vi "step4 Solve.vi"(8 "error in (no error)":errorcluster, 11 "cube in":T1) -> (0 "error out":errorcluster, 1 "upper cross solved?":bool, 3 "cube out":T1)   [LabVIEW 2011]
doc: "Rotate cube as necessary so that the top middle piece matches the desired start colour.\n\nNo transformations are done in this VI, the operations are loaded on the the operation queue bus."
uses:
  Typedef/cube.ctl
  Typedef/face.ctl
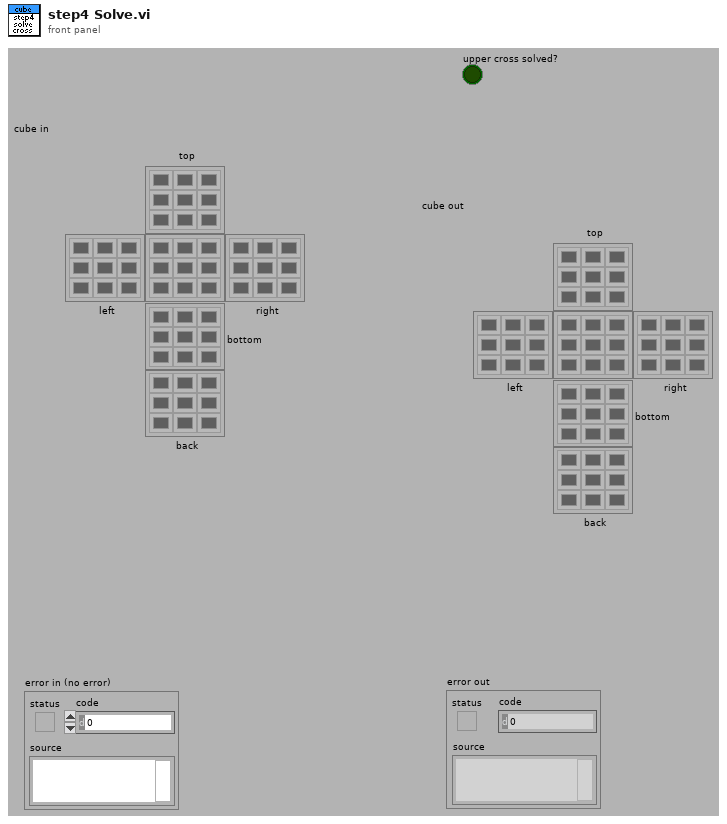
[diagram p1: front panel]
types:
  T1 = typedef "cube.ctl" = cluster{"top":T2, "left":T2, "right":T2, "bottom":T2, "back":T2, "front":T2}
  T2 = typedef "face.ctl" = u32[][]
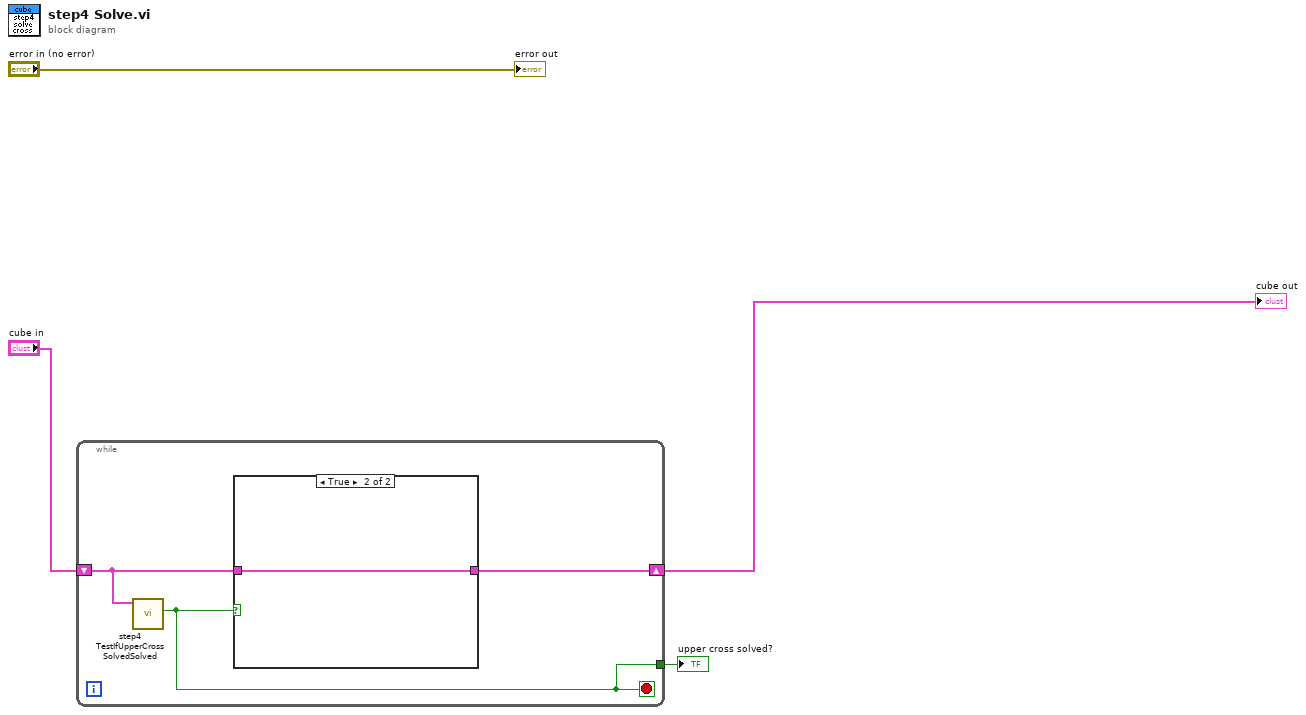
[diagram p0: block diagram]
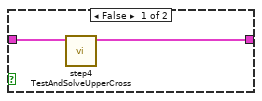
[diagram p2: hidden frame]
diagram:
  n1 = while {
    shift-right: [w6] -> w3
    shift-left: "cube in" -> [w7]
    tunnel: [w5] -> w2
    stop <- w5 stop-if-true
    n2 = call "step4 TestIfUpperCrossSolvedSolved.vi"("cube in"=w7) -> ("upper cross solved?"=w5:bool)  [unwired: 9 in, 1 out]
    n3 = case shown="True" w5 {
      tunnel: w7 -> [w9 w10]
      tunnel: [w8 w10] -> w6
      frame False {
        n4 = call "step4 TestAndSolveUpperCross.vi"("cube in"=w9) -> ("cube out"=w8:T1)  [unwired: 10 in]
      }
      frame True {
      }
    }
  }
  "upper cross solved?" <- w2
  "cube out" <- w3
  "error out" <- "error in (no error)"
